vi "Pre Launch Init.vi"(11 "Camera Controller in":refnum<class "Camera Controller.lvclass">) -> (0 "error out":errorcluster, 3 "Camera Controller out":refnum<class "Camera Controller.lvclass">)   [LabVIEW 2019, in "Camera Controller.lvlib" / "Camera Controller.lvclass"]
doc: "(<B>Filename</B>: Actor Framework.lvlib:Actor.lvclass:Pre Launch Init.vi)\n\nDefines behavior that occurs after the Launch Nested Actor method is invoked but before the actor's Actor Core method begins running.\n\nBy default, this method does nothing. A descendant class may override it to define behavior."
uses:
  Camera Controller.lvclass
  <vilib>/ActorFramework/Message Enqueuer/Message Enqueuer.lvclass
  <vilib>/vision/Image Controls.llb/IMAQ Image.ctl
  <vilib>/ActorFramework/Actor/Actor.lvclass
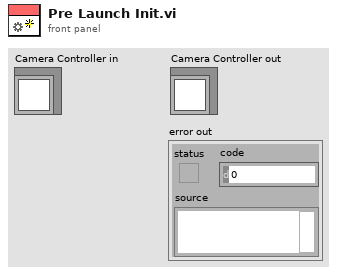
[diagram p1: front panel]
types:
  T1 = cluster{"Camera Id":i32, "Camera Name":string, "Exposure Time":i32, "AOI":i32[]}
  T2 = cluster{"State":string, "Image File path":cluster{"Path":path, "Camera ID":i32}[]}
  T3 = typedef "IMAQ Image.ctl" = refnum<image>
  T4 = cluster{"Image out":T3, "Camera Location":string, "Count":u64, "RecieverSequence":cluster{"RecieverID":dbl, "Index":dbl}[]}
  T5 = cluster{"Nested Actor enqueuer":refnum<class "Message Enqueuer.lvclass">, "Actor Name":string}
  T6 = cluster{"Light Camera Name":string, "Status":string}
  T7 = cluster{"Reciever Enqueuers":refnum<class "Message Enqueuer.lvclass">, "Reciever Name":string, "Reciever ID":i32}
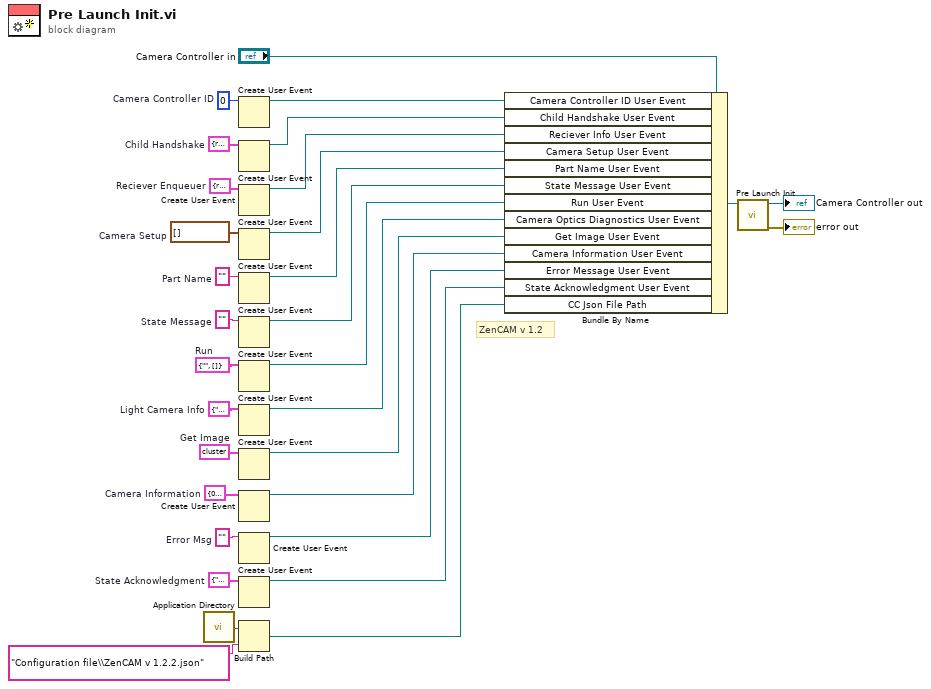
[diagram p0: block diagram]
diagram:
  w2 = T1 {"Camera Id"=0, "Camera Name"="", "Exposure Time"=0, "AOI"=[]}  # Camera Information
  w19 = cluster{"State":string, "Status":string} {"State"="", "Status"=""}  # State Acknowledgment
  w20 = ""  # Error Msg
  w21 = T2 {"State"="", "Image File path"=[]}  # Run
  w22 = T4 {"Image out"=refnum, "Camera Location"="", "Count"=0, "RecieverSequence"=[{"RecieverID"=0.0, "Index"=1.0}, {"RecieverID"=1.0, "Index"=2.0}]}  # Get Image
  w23 = T5 {"Nested Actor enqueuer"=refnum, "Actor Name"=""}  # Child Handshake
  w24 = T6 {"Light Camera Name"="", "Status"=""}  # Light Camera Info
  w25 = ""  # Part Name
  w26 = ""  # State Message
  w27 = cluster{"Camera ID":i32, "Exposure time":i32}[] []  # Camera Setup
  w28 = 0  # Camera Controller ID
  w29 = T7 {"Reciever Enqueuers"=refnum, "Reciever Name"="", "Reciever ID"=0}  # Reciever Enqueuer
  # "ZenCAM v 1.2"
  n1 = call <vilib>:"Application Directory.vi"() -> ("Application Directory"=w18:path)
  n2 = Create User Event(user event datatype=w28) -> (user event=w16:refnum<user-event>)  [unwired: 1 in, 1 out]
  n3 = Create User Event(user event datatype=w23) -> (user event=w15:refnum<user-event>)  [unwired: 1 in, 1 out]
  n4 = Create User Event(user event datatype=w29) -> (user event=w3:refnum<user-event>)  [unwired: 1 in, 1 out]
  n5 = Create User Event(user event datatype=w27) -> (user event=w14:refnum<user-event>)  [unwired: 1 in, 1 out]
  n6 = Create User Event(user event datatype=w25) -> (user event=w13:refnum<user-event>)  [unwired: 1 in, 1 out]
  n7 = Create User Event(user event datatype=w26) -> (user event=w12:refnum<user-event>)  [unwired: 1 in, 1 out]
  n8 = Create User Event(user event datatype=w21) -> (user event=w11:refnum<user-event>)  [unwired: 1 in, 1 out]
  n9 = Create User Event(user event datatype=w24) -> (user event=w10:refnum<user-event>)  [unwired: 1 in, 1 out]
  n10 = Create User Event(user event datatype=w22) -> (user event=w9:refnum<user-event>)  [unwired: 1 in, 1 out]
  n11 = Create User Event(user event datatype=w2) -> (user event=w1:refnum<user-event>)  [unwired: 1 in, 1 out]
  n12 = Create User Event(user event datatype=w20) -> (user event=w8:refnum<user-event>)  [unwired: 1 in, 1 out]
  n13 = Create User Event(user event datatype=w19) -> (user event=w7:refnum<user-event>)  [unwired: 1 in, 1 out]
  n14 = Build Path(base path=w18, name or relative path="Configuration file\\ZenCAM v 1.2.2.json") -> (appended path=w6:path)
  n15 = Bundle By Name(cluster="Camera Controller in", "Camera Controller ID User Event"=w16, "Child Handshake User Event"=w15, "Reciever Info User Event"=w3, "Camera Setup User Event"=w14, "Part Name User Event"=w13, "State Message User Event"=w12, "Run User Event"=w11, "Camera Optics Diagnostics User Event"=w10, "Get Image User Event"=w9, "Camera Information User Event"=w1, "Error Message User Event"=w8, "State Acknowledgment User Event"=w7, "CC Json File Path"=w6) -> (w4:refnum<class "Camera Controller.lvclass">)
  n16 = call-parent "Pre Launch Init.vi"("Actor in"=w4) -> ("error out"=→"error out":errorcluster, "Actor out"=→"Camera Controller out":refnum<class "Camera Controller.lvclass">)  [unwired: 9 in]
